vi "Write BatchData.vi"(8 "error in (no error)":errorcluster, 10 "BatchData":refnum<vi>, 11 "RSeries_CAM in":refnum<class "RSeries_CAM.lvclass">) -> (0 "error out":errorcluster, 3 "RSeries_CAM out":refnum<class "RSeries_CAM.lvclass">)   [LabVIEW 2024, in "RSeries_CAM.lvlib" / "RSeries_CAM.lvclass"]
uses:
  RSeries_CAM.lvclass
  CTRLS/Open Batch Data.ctl
  RSeries_CAM.lvclass/RSeries_CAM.ctl
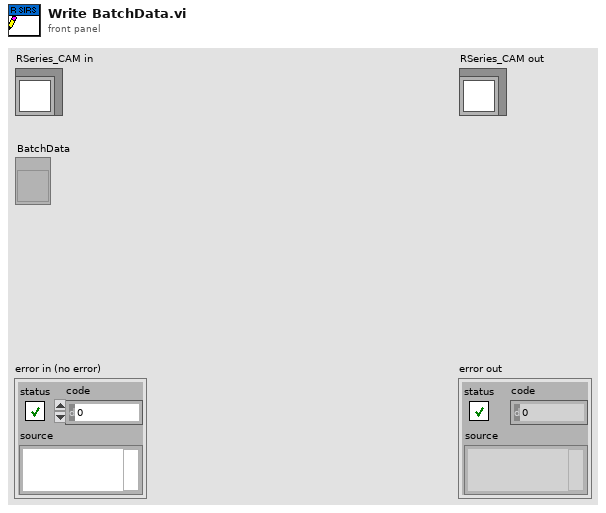
[diagram p1: front panel]
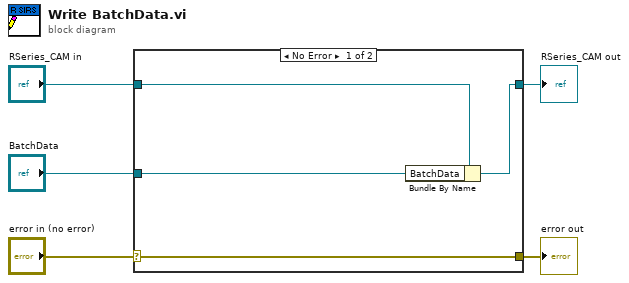
[diagram p0: block diagram]
diagram:
  n1 = case shown="No Error" "error in (no error)" {
    selector: "error in (no error)" -> [w9 w10]
    tunnel: [w9 w10] -> w4
    tunnel: [w7 w11] -> w2
    tunnel: "RSeries_CAM in" -> [w8 w11]
    tunnel: "BatchData" -> [w6 _]
    frame No Error {
      n2 = Bundle By Name(cluster=w8, "BatchData"=w6) -> (w7:refnum<class "RSeries_CAM.lvclass">)
    }
    frame Error {
    }
  }
  "error out" <- w4
  "RSeries_CAM out" <- w2
